vi "Timez.vi"() -> ()   [LabVIEW 2012]
uses:
  <vilib>/express/express analysis/Spectral/Block/exnSpectralBlock spectral measurements PSD poly.vi
  <vilib>/express/express analysis/Spectral/Block/exnSpectralBlock spectral measurements PSD DDT.vi
  <vilib>/express/express analysis/Spectral/XNode/ExpressSpectralMeasurementsBlockNode.xnode
  <vilib>/gmath/NI_Gmath.lvlib
panel:
  out "CI":dbl
  out "SFM":dbl
  out "算数平均值":dbl
  out "几何平均值":dbl
  out "归一化":waveform(dbl)(graph)
  out "原始波形":dynamicdata(graph)
  out "带时间信息波形":waveform(dbl)(graph)
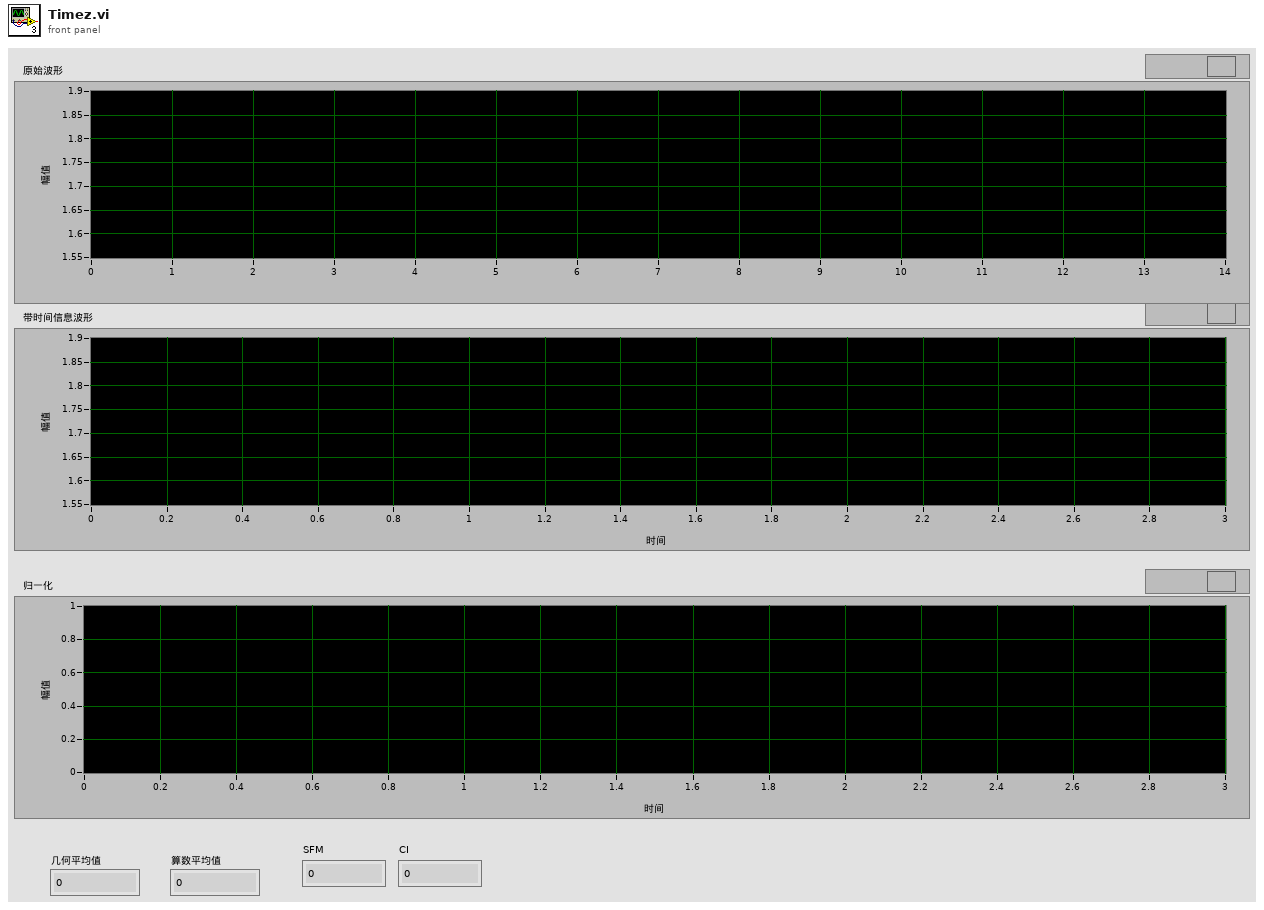
[diagram p1: front panel]
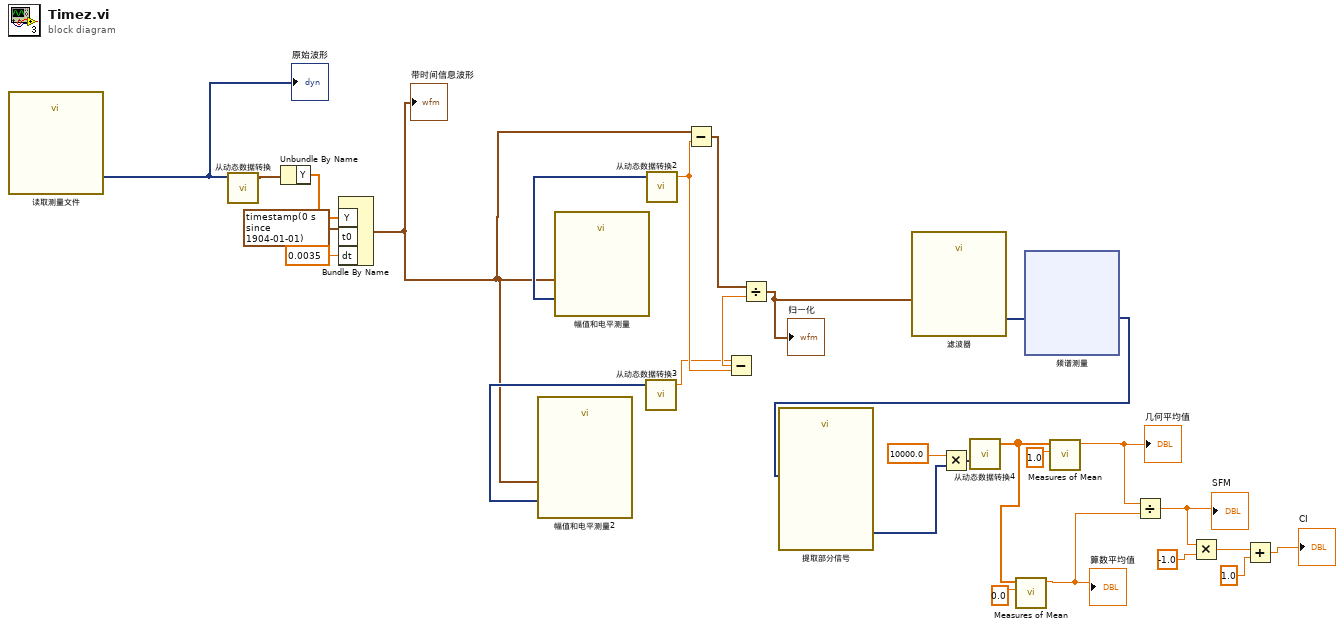
[diagram p0: block diagram]
diagram:
  n1 = call "读取测量文件"() -> ("Signals"=w24:dynamicdata)  [unwired: 6 in, 5 out]
  "原始波形" <- w24
  n2 = call "从动态数据转换"("Dynamic Data Type"=w24) -> ("Waveform"=w25:waveform(dbl))  [unwired: 3 in]
  n3 = Unbundle By Name(w25) -> ("Y"=w28:dbl[])
  n4 = Bundle By Name("Y"=w28, "t0"=timestamp(0 s since 1904-01-01), "dt"=0.0035) -> (w17:waveform(dbl))  [unwired: 1 in]
  "带时间信息波形" <- w17
  n5 = call "幅值和电平测量2"("Signals"=w17) -> ("Positive Peak"=w18:dynamicdata)  [unwired: 13 in, 1 out]
  n6 = call "幅值和电平测量"("Signals"=w17) -> ("Negative Peak"=w19:dynamicdata)  [unwired: 13 in, 1 out]
  n7 = call "从动态数据转换3"("Dynamic Data Type"=w18) -> ("Scalar"=w15:dbl)  [unwired: 3 in]
  n8 = call "从动态数据转换2"("Dynamic Data Type"=w19) -> ("Scalar"=w16:dbl)  [unwired: 3 in]
  n9 = Subtract(x=w17, y=w16) -> (x-y=w20:waveform(dbl))
  n10 = Subtract(x=w15, y=w16) -> (x-y=w23:dbl)
  n11 = Divide(x=w20, y=w23) -> (x/y=w22:waveform(dbl))
  "归一化" <- w22
  n12 = call "滤波器"("Signal"=w22) -> ("Filtered Signal"=w21:dynamicdata)  [unwired: 9 in, 1 out]
  n13 = xnode "频谱测量"("信号"=w21) -> ("PSD"=w14:dynamicdata)  [unwired: 1 in, 1 out]
  n14 = call "提取部分信号"("Signals"=w14) -> ("Section"=w12:dynamicdata)  [unwired: 9 in, 1 out]
  n15 = Multiply(x=10000.0 ("正峰"), y=w12) -> (x*y=w11:dynamicdata)
  n16 = call "从动态数据转换4"("Dynamic Data Type"=w11) -> ("Array"=w9:dbl[])  [unwired: 3 in]
  n17 = call <vilib>:"Measures of Mean.vi"("type"=0.0 ("正峰"), "x array"=w9) -> ("mean value"=w6:dbl)  [unwired: 8 in, 1 out]
  "算数平均值" <- w6
  n18 = call <vilib>:"Measures of Mean.vi"("type"=1.0 ("正峰"), "x array"=w9) -> ("mean value"=w7:dbl)  [unwired: 8 in, 1 out]
  "几何平均值" <- w7
  n19 = Divide(x=w7, y=w6) -> (x/y=w4:dbl)
  "SFM" <- w4
  n20 = Multiply(x=w4, y=-1.0 ("正峰")) -> (x*y=w2:dbl)
  n21 = Add(x=w2, y=1.0 ("正峰")) -> (x+y=→"CI":dbl)
